vi "expand bundle.vi"(8 "error in (no error)":errorcluster, 10 "Results from processing ref in":refnum<vi>, 11 "VI Refnum":refnum<vi>) -> (0 "error out":errorcluster, 2 "Bundle ref out":refnum<vi>)   [LabVIEW 2013]
uses:
  <vilib>/Utility/traverseref.llb/TRef TravTarget.ctl
  <vilib>/Utility/traverseref.llb/VI Scripting - Traverse.lvlib
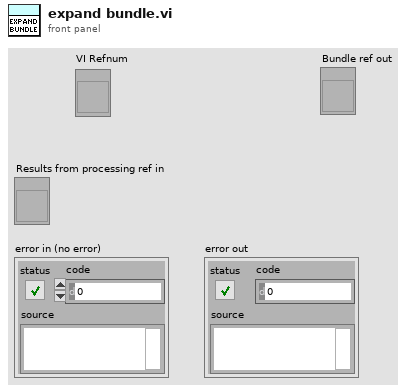
[diagram p1: front panel]
types:
  T1 = typedef "TRef TravTarget.ctl" = enum16{"FP", "BD", "Other"}
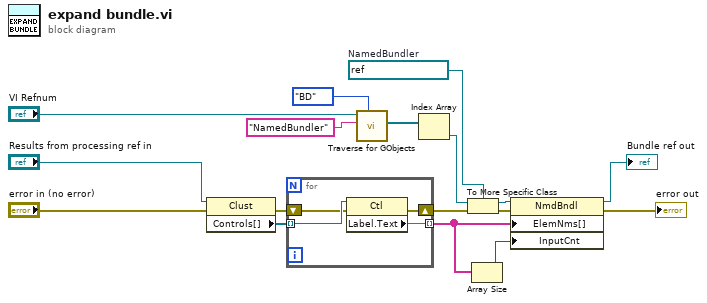
[diagram p0: block diagram]
diagram:
  w13 = refnum<vi> refnum  # NamedBundler
  n1 = property class="Clust"(reference="Results from processing ref in", error in="error in (no error)") -> (error out=w14:errorcluster, "Controls[]"=w12:refnum<vi>[])  [unwired: 1 out]
  n2 = for {
    tunnel: w12 -> [w21] mode=indexing
    tunnel: [w20] -> w2 mode=indexing
    shift-right: [w18] -> w15
    shift-left: w14 -> [w19]
    n3 = property class="Ctl"(reference=w21, error in=w19) -> (error out=w18:errorcluster, "Label.Text"=w20:string)  [unwired: 1 out]
  }
  n4 = call <vilib>:"Traverse for GObjects.vi"("Traverse Target"=TRef_TravTarget."BD", "Class Name"="NamedBundler", "VI Refnum"="VI Refnum") -> ("References"=w10:refnum<vi>[])  [unwired: 5 in, 3 out]
  n5 = Index Array(array=w10) -> (element=w7:refnum<vi>)  [unwired: 1 in]
  n6 = To More Specific Class(target class=w13, reference=w7, error in=w15) -> (specific class reference=w11:refnum<vi>, error out=w16:errorcluster)
  n7 = Array Size(array=w2) -> (size(s)=w1:i32)
  n8 = property class="NmdBndl"(reference=w11, error in=w16, "ElemNms[]"=w2, "InputCnt"=w1) -> (reference out=→"Bundle ref out":refnum<vi>, error out=→"error out":errorcluster)
